vi "Uarm_Right_Hand_Follow.vi"(7 "Boundary":T2={"X max"=310.0, "X min"=147.0, "Z max"=148.0, "Z min"=-92.0}, 8 "error in":errorcluster, 9 "full read buffer in":string, 10 "Calibrated Oculus Data":T1, 11 "Machine In":refnum<visa-resource-name>) -> (0 "error out":errorcluster, 1 "full read buffer out":string, 3 "Machine Out":refnum<visa-resource-name>)   [LabVIEW 2017]
uses:
  Calibrated Oculus Data.ctl
panel:
  in  "Gripper Closed":bool
  in  "Z-Position":dbl
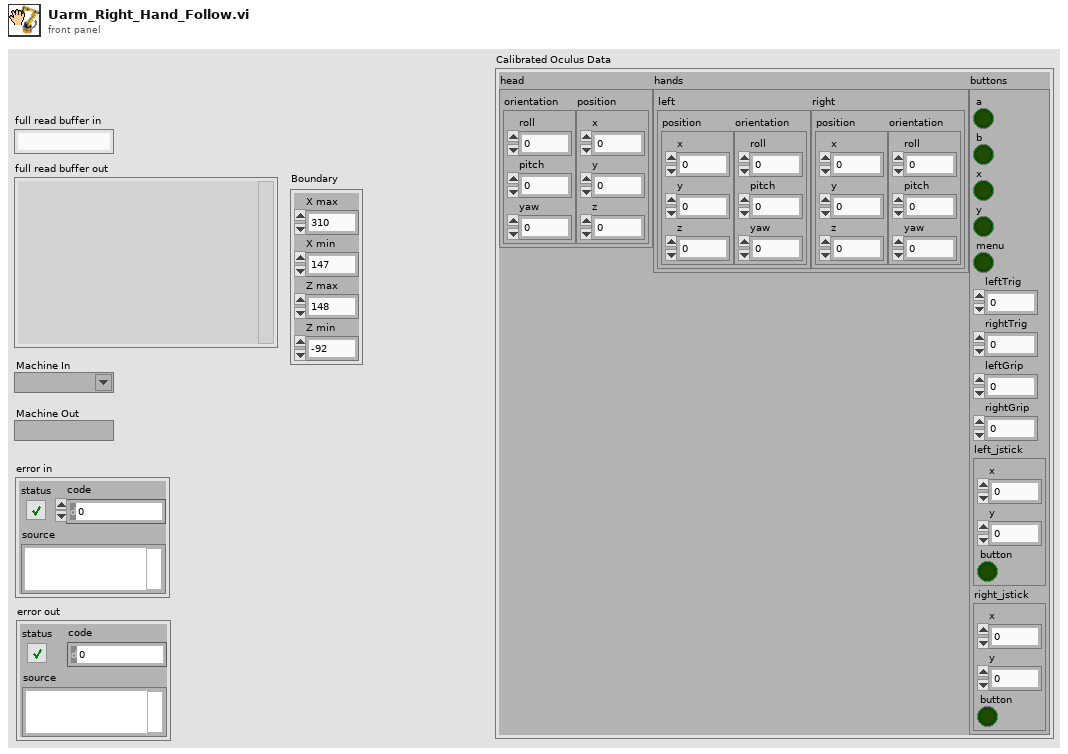
[diagram p1: front panel]
types:
  T1 = typedef "Calibrated Oculus Data.ctl" = cluster{"head":cluster{"orientation":cluster{"roll":dbl, "pitch":dbl, "yaw":dbl}, "position":cluster{"x":dbl, "y":dbl, "z":dbl}}, "hands":cluster{"left":cluster{"position":cluster{"x":dbl, "y":dbl, "z":dbl}, "orientation":cluster{"roll":dbl, "pitch":dbl, "yaw":dbl}}, "right":cluster{"position":cluster{"x":dbl, "y":dbl, "z":dbl}, "orientation":cluster{"roll":dbl, "pitch":dbl, "yaw":dbl}}}, "buttons":cluster{"a":bool, "b":bool, "x":bool, "y":bool, "menu":bool, "leftTrig":dbl, "rightTrig":dbl, "leftGrip":dbl, "rightGrip":dbl, "left_jstick":cluster{"x":dbl, "y":dbl, "button":bool}, "right_jstick":cluster{"x":dbl, "y":dbl, "button":bool}}}
  T2 = cluster{"X max":dbl, "X min":dbl, "Z max":dbl, "Z min":dbl}
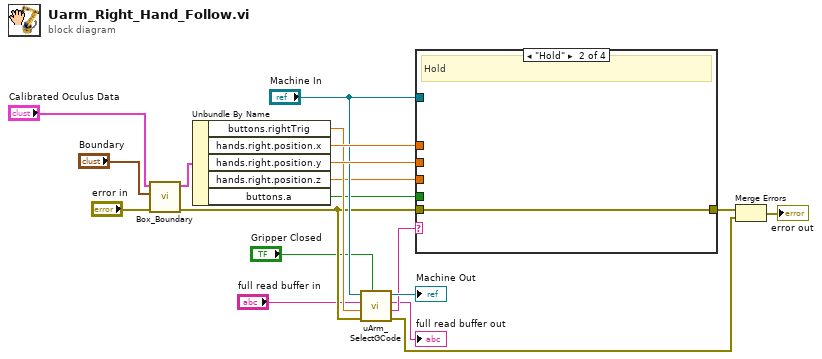
[diagram p0: block diagram]
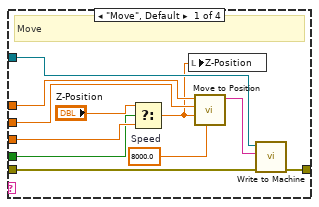
[diagram p2: hidden frame]
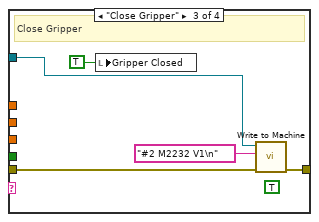
[diagram p3: hidden frame]
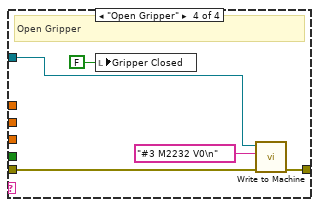
[diagram p4: hidden frame]
diagram:
  n1 = call "Box_Boundary.vi"("error in"="error in", "Boundary"="Boundary", "Calibrated Oculus Data"="Calibrated Oculus Data") -> ("error out"=w9:errorcluster, "Calibrated Oculus Data 2"=w11:T1)  [unwired: 7 in]
  n2 = Unbundle By Name(w11) -> ("buttons.rightTrig"=w17:dbl, "hands.right.position.x"=w19:dbl, "hands.right.position.y"=w18:dbl, "hands.right.position.z"=w12:dbl, "buttons.a"=w7:bool)
  n3 = call "uArm_SelectGCode.vi"("Gripper Closed"="Gripper Closed", "error in (no error)"=w9, "rightTrig"=w17, "full read buffer in"="full read buffer in", "VISA Refnum in"="Machine In") -> ("error out"=w13:errorcluster, "Command"=w3:string, "full read buffer out"=→"full read buffer out":string, "VISA Refnum out"=→"Machine Out":refnum<visa-resource-name>)  [unwired: 3 in]
  n4 = case shown="\"Hold\"" w3 {
    tunnel: w19 -> [w29 _ _ _]
    tunnel: w18 -> [w28 _ _ _]
    tunnel: w9 -> [w25 w31 w34 w38]
    tunnel: [w27 w31 w33 w37] -> w14
    tunnel: "Machine In" -> [w24 _ w35 w40]
    tunnel: w12 -> [w21 _ _ _]
    tunnel: w7 -> [w20 _ _ _]
    frame "Move", Default {
      w30 = 8000.0  # Speed
      # "Move"
      n5 = Select(t="Z-Position", s=w20, f=w21) -> (s? t:f=w22:dbl)
      n6 = local write "Z-Position"(w22) -> ()
      n7 = call "Move to Position.vi"("Speed"=w30, "Z-Position"=w22, "Y-Position"=w28, "X-Position"=w29) -> ("G-Code String"=w26:string)  [unwired: 7 in]
      n8 = call "Write to Machine .vi"("error in (no error)"=w25, "G-Code String In"=w26, "Machine In"=w24) -> ("error out"=w27:errorcluster)  [unwired: 7 in, 1 out]
    }
    frame "Hold" {
      # "Hold"
    }
    frame "Close Gripper" {
      (unwired) TRUE
      # "Close Gripper"
      n9 = local write "Gripper Closed"(TRUE) -> ()
      n10 = call "Write to Machine .vi"("error in (no error)"=w34, "G-Code String In"="#2 M2232 V1\n", "Machine In"=w35) -> ("error out"=w33:errorcluster)  [unwired: 7 in, 1 out]
    }
    frame "Open Gripper" {
      # "Open Gripper"
      n11 = local write "Gripper Closed"(FALSE ("Gripper Closed")) -> ()
      n12 = call "Write to Machine .vi"("error in (no error)"=w38, "G-Code String In"="#3 M2232 V0\n", "Machine In"=w40) -> ("error out"=w37:errorcluster)  [unwired: 7 in, 1 out]
    }
  }
  n13 = Merge Errors(w14, w13) -> (→"error out":errorcluster)
